vi "AutoPlayLoad.vi"(1 "Selected Auto Play":u16, 2 "Available Auto Plays":string[](array[string])) -> (0 "Loaded Auto Play":string)   [LabVIEW 2023]
doc: "This VI reads the selected autonomous play text file from the roboRIO file system."
uses:
  <vilib>/Utility/error.llb/Trim Whitespace One-Sided.vi
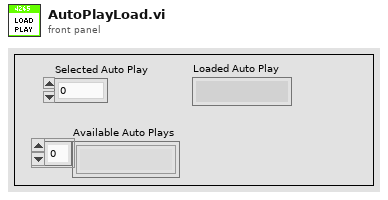
[diagram p1: front panel]
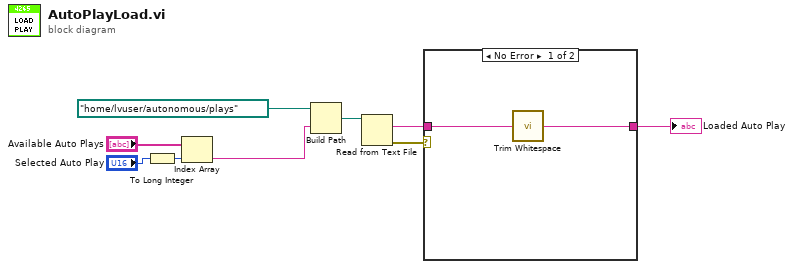
[diagram p0: block diagram]
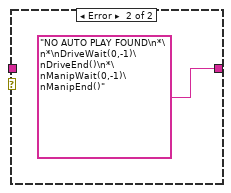
[diagram p2: hidden frame]
diagram:
  n1 = To Long Integer(number="Selected Auto Play") -> (32bit integer=w5:i32)
  n2 = Index Array(array="Available Auto Plays", index=w5) -> (element=w6:string)
  n3 = Build Path(base path=path "/home/lvuser/autonomous/plays" ("path"), name or relative path=w6) -> (appended path=w4:path)
  n4 = Read from Text File(file (use dialog)=w4) -> (text=w2:string, error out=w3:errorcluster)  [unwired: 3 in, 2 out]
  n5 = case shown="No Error" w3 {
    tunnel: w2 -> [w10 _]
    tunnel: [w11 "NO AUTO PLAY FOUND\n*\n*\nDriveWait(0,-1)\nDriveEnd()\n*\nManipWait(0,-1)\nManipEnd()"] -> w1
    frame No Error {
      n6 = call <vilib>:"Trim Whitespace.vi"("string"=w10) -> ("trimmed string"=w11:string)  [unwired: 1 in]
    }
    frame Error {
    }
  }
  "Loaded Auto Play" <- w1
